vi "exp3.vi"() -> ()   [LabVIEW 2014]
uses:
  <vilib>/Analysis/NI_AALPro.lvlib
panel:
  out "数据":dbl[][](array[numeric])
  in  "开关":bool
  out "待测电阻值":dbl
  in  "时间间隔":dbl[unit]
  in  "标准电阻":dbl
  in  "测量数据点数":dbl
  in  "输出电压步长":dbl[unit]
  out "电阻的伏安特性曲线":cluster{"Y":dbl[], "Y":dbl[]}[](graph)
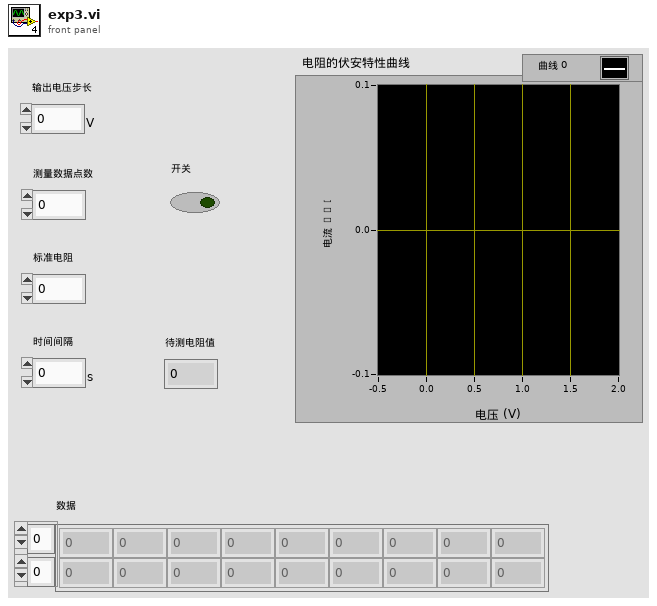
[diagram p1: front panel]
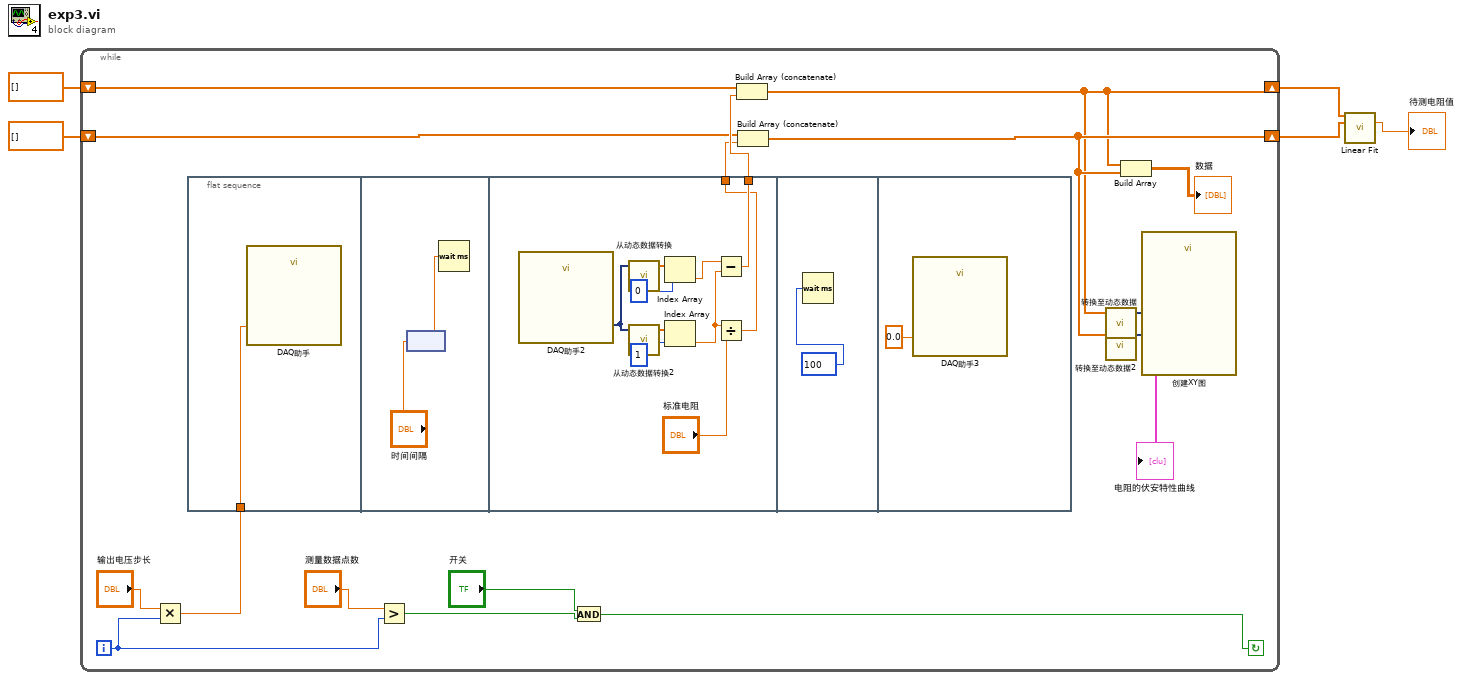
[diagram p0: block diagram]
diagram:
  n1 = while {
    shift-right: [w8] -> w4
    shift-left: dbl[] [] -> [w12]
    shift-right: [w7] -> w5
    shift-left: dbl[] [] -> [w11]
    i -> [w18]
    stop <- w15 continue-if-true
    n2 = Multiply(x="输出电压步长", y=w18) -> (x*y=w20:dbl[unit])
    n3 = flat-sequence {
      tunnel: w20 -> [w23]
      tunnel: [w27] -> w14
      tunnel: [w26] -> w13
      frame #0 {
        n4 = call "DAQ助手"("data"=w23) -> ()  [unwired: 17 in, 2 out]
      }
      frame #1 {
        n5 = node("时间间隔") -> (w24:dbl)
        n6 = Wait (ms)(milliseconds to wait=w24) -> ()  [unwired: 1 out]
      }
      frame #2 {
        n7 = call "DAQ助手2"() -> ("data"=w34:dynamicdata)  [unwired: 17 in, 2 out]
        n8 = call "从动态数据转换"("Dynamic Data Type"=w34) -> ("Array"=w35:dbl[])  [unwired: 3 in]
        n9 = call "从动态数据转换2"("Dynamic Data Type"=w34) -> ("Array"=w33:dbl[])  [unwired: 3 in]
        n10 = Index Array(array=w35, index=0 ("索引")) -> (element=w30:dbl)
        n11 = Index Array(array=w33, index=1 ("索引")) -> (element=w28:dbl)
        n12 = Subtract(x=w30, y=w28) -> (x-y=w27:dbl)
        n13 = Divide(x=w28, y="标准电阻") -> (x/y=w26:dbl)
      }
      frame #3 {
        n14 = Wait (ms)(milliseconds to wait=u32 100 ("等待时间（毫秒）")) -> ()  [unwired: 1 out]
      }
      frame #4 {
        n15 = call "DAQ助手3"("data"=0.0 ("数据")) -> ()  [unwired: 17 in, 2 out]
      }
    }
    n16 = Greater?(x="测量数据点数", y=w18) -> (0:w16:bool)
    n17 = And(x="开关", y=w16) -> (x .and. y?=w15:bool)
    n18 = Build Array (concatenate)(w11, w14) -> (w7:dbl[])
    n19 = Build Array (concatenate)(w12, w13) -> (w8:dbl[])
    n20 = call "转换至动态数据"("Array"=w7) -> ("Dynamic Data Type"=w10:dynamicdata)  [unwired: 3 in]
    n21 = call "转换至动态数据2"("Array"=w8) -> ("Dynamic Data Type"=w9:dynamicdata)  [unwired: 3 in]
    n22 = Build Array(w7, w8) -> (→"数据":dbl[][])
    n23 = call "创建XY图"("Y Input"=w9, "X Input"=w10) -> ("XY Graph"=→"电阻的伏安特性曲线":cluster{"X":dbl[], "Y":dbl[]}[])  [unwired: 8 in, 1 out]
  }
  n24 = call <vilib>:"Linear Fit.vi"("Y"=w5, "X"=w4) -> ("slope"=→"待测电阻值":dbl)  [unwired: 9 in, 4 out]
